vi "get_op_no.vi"(8 "error in (no error)":errorcluster, 11 "SsaId in":refnum<class "SsaId.lvclass">) -> (0 "error out":errorcluster, 1 "is_set?":bool, 2 "op_no":T1, 3 "SsaId out":refnum<class "SsaId.lvclass">)   [LabVIEW 2020, in "mlir.lvlib" / "SsaId.lvclass"]
uses:
  SsaId.lvclass
  op_no.ctl
  SsaId.lvclass/SsaId.ctl
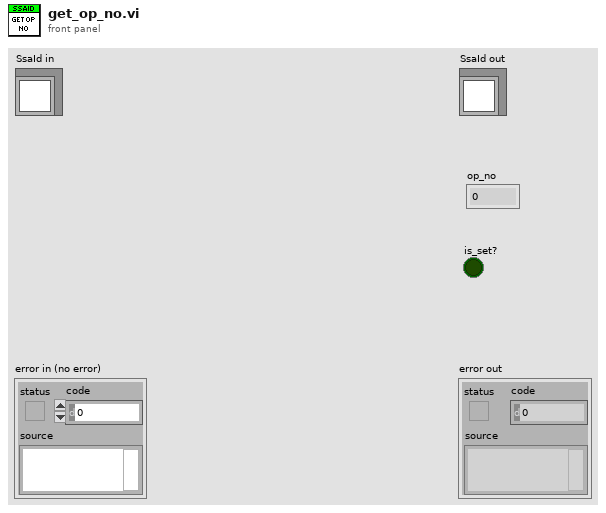
[diagram p1: front panel]
types:
  T1 = typedef "mlir.lvlib/SsaId.lvclass/op_no.ctl" = u32
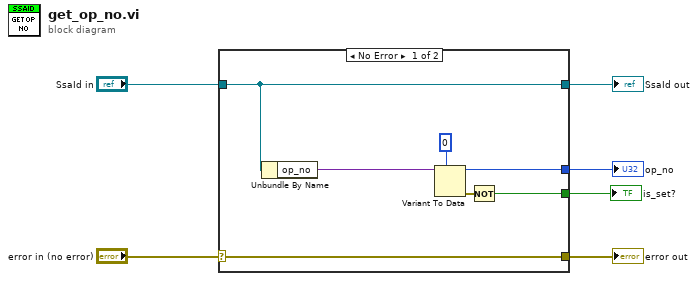
[diagram p0: block diagram]
diagram:
  n1 = case shown="No Error" "error in (no error)" {
    selector: "error in (no error)" -> [w13 w14]
    tunnel: [w13 w14] -> w5
    tunnel: [w12 w15] -> w3
    tunnel: "SsaId in" -> [w12 w15]
    tunnel: [w9 _] -> w2
    tunnel: [w7 _] -> w1
    frame No Error {
      n2 = Unbundle By Name(w12) -> ("op_no"=w11:variant)
      n3 = Variant To Data(type=T1 0 ("op_no"), Variant=w11) -> (data=w9:T1, error out=w8:errorcluster)  [unwired: 1 in]
      n4 = Not(x=w8) -> (.not. x?=w7:bool)
    }
    frame Error {
    }
  }
  "error out" <- w5
  "SsaId out" <- w3
  "op_no" <- w2
  "is_set?" <- w1
